vi "Global.vi"() -> ()   [LabVIEW 2016, in "Agilent 415X Series.lvlib"]
uses:
  Agilent 415X Series.lvlib
panel:
  in  "system setting":T1(array[cluster])
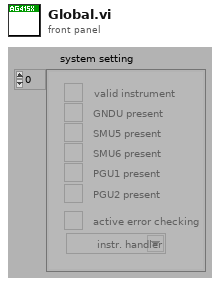
[diagram p1: front panel]
types:
  T1 = cluster{"valid instrument":bool, "GNDU present":bool, "SMU5 present":bool, "SMU6 present":bool, "PGU1 present":bool, "PGU2 present":bool, "active error checking":bool, "instr. handler":refnum<visa-resource-name>}[]
diagram:
